vi "Match string counter.vi"(8 "error in (no error)":errorcluster, 10 "Match String":string, 11 "Input string":string) -> (0 "error out":errorcluster, 3 "Count":i32)   [LabVIEW 2014]
doc: "This VI takes the string as input and finds how many times the \"Match string\" appears in it.\n\nDesigned by HB\nhaba@dtu.dk"
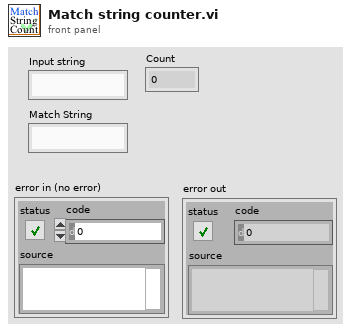
[diagram p1: front panel]
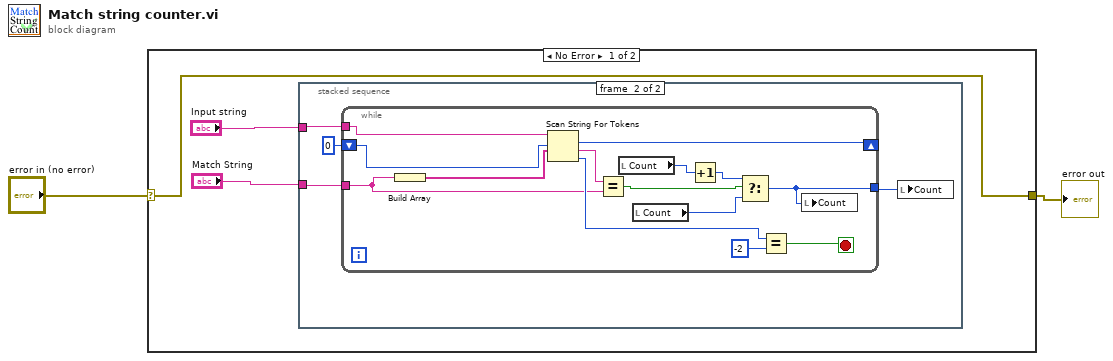
[diagram p0: block diagram]
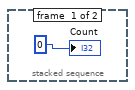
[diagram p2: hidden frame]
diagram:
  n1 = case shown="No Error" "error in (no error)" {
    selector: "error in (no error)" -> [w3 w25]
    tunnel: [w3 w25] -> w1
    frame No Error {
      n2 = stacked-sequence {
        tunnel: "Input string" -> [_ w10]
        tunnel: "Match String" -> [_ w9]
        frame #0 {
          "Count" <- 0 ("Count")
        }
        frame #1 {
          n3 = while {
            shift-right: [w19] -> _
            shift-left: 0 ("offset past token") -> [w18]
            tunnel: [w13] -> w7
            tunnel: w10 -> [w17]
            tunnel: w9 -> [w15]
            stop <- w21 stop-if-true
            n4 = Build Array(w15) -> (w16:string[])
            n5 = Scan String For Tokens(7:w16, 8:w18, 9:w17) -> (0:w20:i32, 1:w23:string, 2:w19:i32)  [unwired: 3 in, 1 out]
            n6 = Equal?(x=w23, y=w15) -> (x = y?=w14:bool)
            n7 = local read "Count"() -> (w12:i32)
            n8 = local read "Count"() -> (w11:i32)
            n9 = Increment(x=w12) -> (x+1=w24:i32)
            n10 = Select(t=w24, s=w14, f=w11) -> (s? t:f=w13:i32)
            n11 = Equal?(x=w20, y=-2) -> (x = y?=w21:bool)
            n12 = local write "Count"(w13) -> ()
          }
          n13 = local write "Count"(w7) -> ()
        }
      }
    }
    frame Error {
    }
  }
  "error out" <- w1
